vi "IRDistanceCalculator.vi"(1 "AIDeviceRef":T1={"DevStatus"={"status"=FALSE, "code"=0, "source"=""}, "Controller"=enum."Controller 1", "Analog Channel"=enum."AI 1"}) -> (0 "Distance(in)":dbl)   [LabVIEW 2014]
uses:
  <vilib>/Rock Robotics/WPI/AnalogChannel/WPI_AnalogChannelDevRef.ctl
  <vilib>/Rock Robotics/SystemInterfaces/Typedef/FPGA_TypedefAnalogModule.ctl
  <vilib>/Rock Robotics/SystemInterfaces/AI/FPGA_AIChannel.ctl
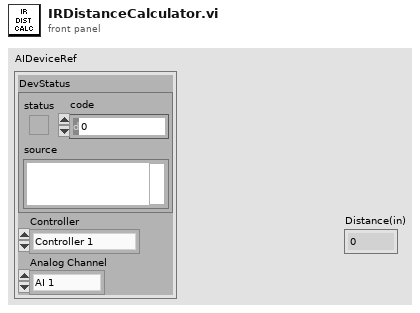
[diagram p1: front panel]
types:
  T1 = typedef "WPI_AnalogChannelDevRef.ctl" = cluster{"DevStatus":errorcluster, "Controller":T2, "Analog Channel":T3}
  T2 = typedef "FPGA_TypedefAnalogModule.ctl" = enum16{"Controller 1"}
  T3 = typedef "FPGA_AIChannel.ctl" = enum8{"AI 0", "AI 1", "AI 2", "AI 3", "AI MXP 0", "AI MXP 1", "AI MXP 2", "AI MXP 3", "Invalid"}
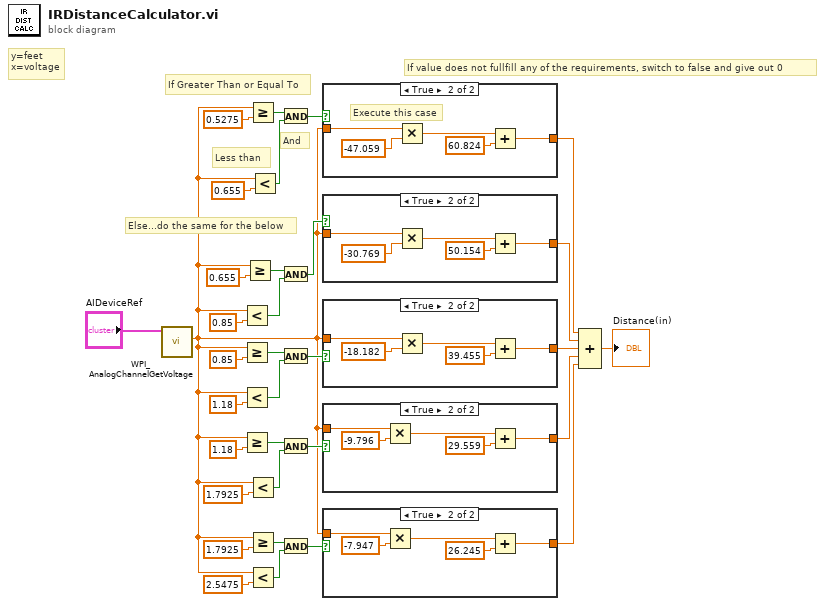
[diagram p0: block diagram]
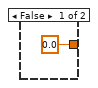
[diagram p2: hidden frame]
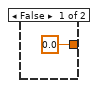
[diagram p3: hidden frame]
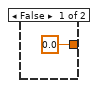
[diagram p4: hidden frame]
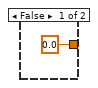
[diagram p5: hidden frame]
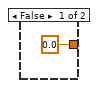
[diagram p6: hidden frame]
diagram:
  # "If value does not fullfill any of the requirements, switch to false and give out 0"
  # "Else...do the same for the below"
  # "Less than"
  # "And"
  # "If Greater Than or Equal To"
  # "y=feet\nx=voltage"
  n1 = call <vilib>:"WPI_AnalogChannelGetVoltage.vi"("AIDeviceRef"="AIDeviceRef") -> ("Voltage"=w3:dbl)  [unwired: 8 in, 2 out]
  n2 = Less?(x=w3, y=0.85) -> (x < y?=w23:bool)
  n3 = Greater Or Equal?(x=w3, y=0.85) -> (x >= y?=w18:bool)
  n4 = Less?(x=w3, y=1.18) -> (x < y?=w17:bool)
  n5 = Greater Or Equal?(x=w3, y=1.18) -> (x >= y?=w12:bool)
  n6 = Greater Or Equal?(x=w3, y=0.655) -> (x >= y?=w24:bool)
  n7 = Greater Or Equal?(x=w3, y=0.5275) -> (x >= y?=w30:bool)
  n8 = Less?(x=w3, y=1.7925) -> (x < y?=w11:bool)
  n9 = Greater Or Equal?(x=w3, y=1.7925) -> (x >= y?=w6:bool)
  n10 = Less?(x=w3, y=2.5475) -> (x < y?=w5:bool)
  n11 = Less?(x=w3, y=0.655) -> (x < y?=w29:bool)
  n12 = And(x=w30, y=w29) -> (x .and. y?=w28:bool)
  n13 = And(x=w24, y=w23) -> (x .and. y?=w21:bool)
  n14 = And(x=w18, y=w17) -> (x .and. y?=w16:bool)
  n15 = And(x=w12, y=w11) -> (x .and. y?=w10:bool)
  n16 = And(x=w6, y=w5) -> (x .and. y?=w4:bool)
  n17 = case shown="True" w28 {
    tunnel: w3 -> [_ w39]
    tunnel: [0.0 w35] -> w27
    frame False {
    }
    frame True {
      # "Execute this case"
      n18 = Multiply(x=w39, y=-47.059) -> (x*y=w37:dbl)
      n19 = Add(x=w37, y=60.824) -> (x+y=w35:dbl)
    }
  }
  n20 = case shown="True" w21 {
    tunnel: [0.0 w42] -> w22
    tunnel: w3 -> [_ w41]
    frame False {
    }
    frame True {
      n21 = Multiply(x=w41, y=-30.769) -> (x*y=w44:dbl)
      n22 = Add(x=w44, y=50.154) -> (x+y=w42:dbl)
    }
  }
  n23 = case shown="True" w16 {
    tunnel: [0.0 w48] -> w15
    tunnel: w3 -> [_ w47]
    frame False {
    }
    frame True {
      n24 = Multiply(x=w47, y=-18.182) -> (x*y=w50:dbl)
      n25 = Add(x=w50, y=39.455) -> (x+y=w48:dbl)
    }
  }
  n26 = case shown="True" w10 {
    tunnel: [0.0 w54] -> w9
    tunnel: w3 -> [_ w53]
    frame False {
    }
    frame True {
      n27 = Multiply(x=w53, y=-9.796) -> (x*y=w56:dbl)
      n28 = Add(x=w56, y=29.559) -> (x+y=w54:dbl)
    }
  }
  n29 = case shown="True" w4 {
    tunnel: [0.0 w60] -> w2
    tunnel: w3 -> [_ w59]
    frame False {
    }
    frame True {
      n30 = Multiply(x=w59, y=-7.947) -> (x*y=w62:dbl)
      n31 = Add(x=w62, y=26.245) -> (x+y=w60:dbl)
    }
  }
  n32 = Compound Arithmetic op=ADD(w27, w22, w15, w9, w2) -> (→"Distance(in)":dbl)
